vi "Preset LOT NUMBER validator.vi"(8 "error in (no error)":errorcluster, 10 "LOT number":string, 11 "VISA resource in":refnum<visa-resource-name>) -> (0 "error out":errorcluster, 3 "VISA resource out":refnum<visa-resource-name>)   [LabVIEW 2025]
uses:
  Preset Number States--enum.ctl
panel:
  # "Set LOT number with validation"
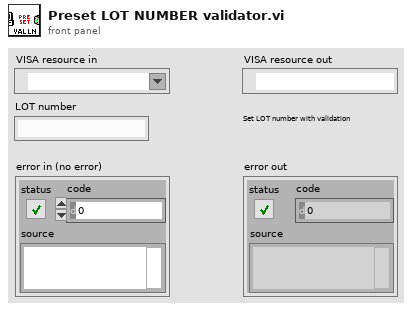
[diagram p1: front panel]
types:
  T1 = typedef "Preset Number States--enum.ctl" = enum16{"Initialize", "Check <=UL", "Check >=LL", "Truncate string", "Send command", "Shutdown"}
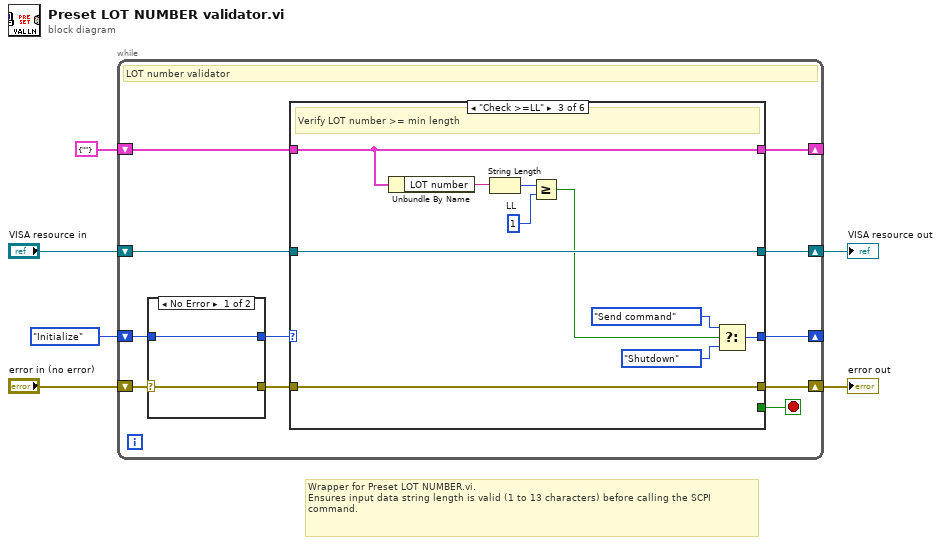
[diagram p0: block diagram]
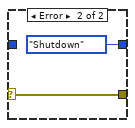
[diagram p2: hidden frame]
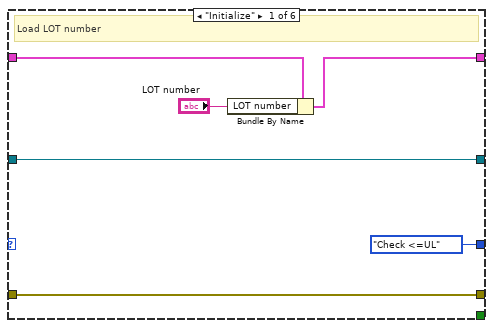
[diagram p3: hidden frame]
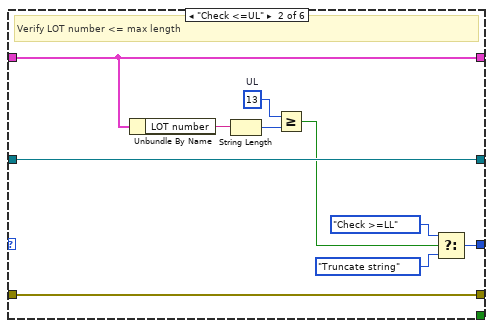
[diagram p4: hidden frame]
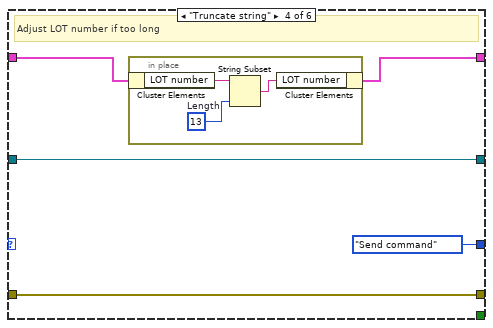
[diagram p5: hidden frame]
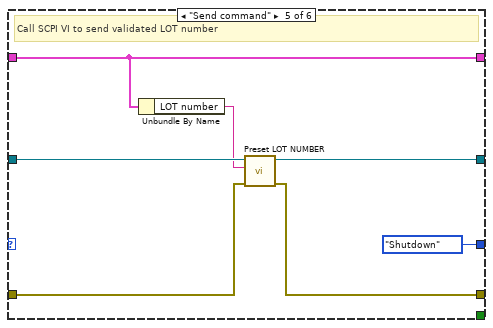
[diagram p6: hidden frame]
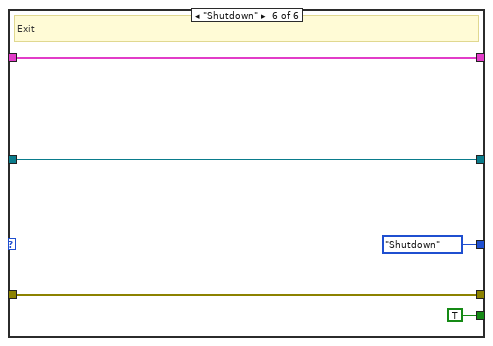
[diagram p7: hidden frame]
diagram:
  # "Wrapper for Preset LOT NUMBER.vi.\nEnsures input data string length is valid (1 to 13 characters) before calling the SCPI command."
  n1 = while {
    shift-right: [w14] -> _
    shift-left: Preset_Number_States--enum."Initialize" -> [w13]
    shift-right: [w8] -> _
    shift-left: cluster{"LOT number":string} {"LOT number"=""} -> [w15]
    shift-right: [w9] -> w3
    shift-left: "VISA resource in" -> [w12]
    shift-right: [w10] -> w4
    shift-left: "error in (no error)" -> [w16]
    stop <- w7 stop-if-true
    # "LOT number validator"
    n2 = case shown="No Error" w16 {
      selector: w16 -> [w19 w20]
      tunnel: [w19 w20] -> w11
      tunnel: [w18 Preset_Number_States--enum."Shutdown"] -> w17
      tunnel: w13 -> [w18 _]
      frame No Error {
      }
      frame Error {
      }
    }
    n3 = case shown="\"Check >=LL\"" w17 {
      tunnel: w15 -> [w25 w32 w40 w50 w57 w65]
      tunnel: [Preset_Number_States--enum."Check <=UL" w35 w43 Preset_Number_States--enum."Send command" Preset_Number_States--enum."Shutdown" Preset_Number_States--enum."Shutdown"] -> w14
      tunnel: w12 -> [w26 w34 w47 w52 w62 w67]
      tunnel: w11 -> [w27 w33 w46 w51 w61 w66]
      tunnel: [w27 w33 w46 w51 w60 w66] -> w10
      tunnel: [w26 w34 w47 w52 w59 w67] -> w9
      tunnel: [w24 w32 w40 w49 w57 w65] -> w8
      tunnel: [_ _ _ _ _ TRUE] -> w7
      frame "Initialize" {
        # "Load LOT number"
        n4 = Bundle By Name(cluster=w25, "LOT number"="LOT number") -> (w24:cluster{"LOT number":string})
      }
      frame "Check <=UL" {
        w37 = 13  # UL
        # "Verify LOT number <= max length"
        n5 = Unbundle By Name(w32) -> ("LOT number"=w31:string)
        n6 = String Length(string=w31) -> (length=w36:i32)
        n7 = Greater Or Equal?(x=w37, y=w36) -> (x >= y?=w28:bool)
        n8 = Select(t=Preset_Number_States--enum."Check >=LL", s=w28, f=Preset_Number_States--enum."Truncate string") -> (s? t:f=w35:T1)
      }
      frame "Check >=LL" {
        w44 = 1  # LL
        # "Verify LOT number >= min length"
        n9 = Unbundle By Name(w40) -> ("LOT number"=w39:string)
        n10 = String Length(string=w39) -> (length=w45:i32)
        n11 = Greater Or Equal?(x=w45, y=w44) -> (x >= y?=w42:bool)
        n12 = Select(t=Preset_Number_States--enum."Send command" ("f"), s=w42, f=Preset_Number_States--enum."Shutdown") -> (s? t:f=w43:T1)
      }
      frame "Truncate string" {
        # "Adjust LOT number if too long"
        n13 = in-place "In Place Element Structure" {
          w54 = 13  # Length
          n14 = in-place-cluster #1 ("Unbundle / Bundle Elements")(w50) -> ("LOT number"=w55:string)
          n15 = String Subset(string=w55, length (rest)=w54) -> (substring=w53:string)  [unwired: 1 in]
          n16 = in-place-cluster #1 ("Unbundle / Bundle Elements")("LOT number"=w53) -> (w49:cluster{"LOT number":string})
        }
      }
      frame "Send command" {
        # "Call SCPI VI to send validated LOT number"
        n17 = Unbundle By Name(w57) -> ("LOT number"=w56:string)
        n18 = call "Preset LOT NUMBER.vi"("error in (no error)"=w61, "LOT number"=w56, "VISA Refnum in"=w62) -> ("error out"=w60:errorcluster, "VISA Refnum out"=w59:refnum<visa-resource-name>)  [unwired: 7 in]
      }
      frame "Shutdown" {
        # "Exit"
      }
    }
  }
  "error out" <- w4
  "VISA resource out" <- w3
